vi "Test.vi"() -> ()   [LabVIEW 2015, in "App Info.lvlib"]
uses:
  App Info.lvlib
  Core Data.ctl
panel:
  out "Data out":T1
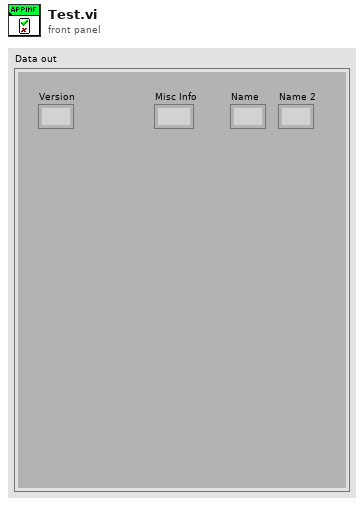
[diagram p1: front panel]
types:
  T1 = typedef "App Info.lvlib/Core Data.ctl" = cluster{"Version":string, "Misc Info":string, "Name":string, "Name 2":string}
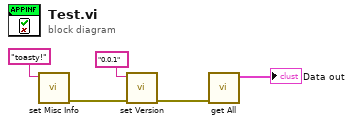
[diagram p0: block diagram]
diagram:
  n1 = call "set Misc Info.vi"("Misc Info"="toasty!") -> ("error out"=w2:errorcluster)  [unwired: 10 in]
  n2 = call "set Version.vi"("error in"=w2, "Version"="0.0.1") -> ("error out"=w1:errorcluster)  [unwired: 9 in]
  n3 = call "get All.vi"("error in"=w1) -> ("Data out"=→"Data out":T1)  [unwired: 9 in, 1 out]
